vi "Timestamp_Analyzer.vi"() -> ()   [LabVIEW 2020]
uses:
  <vilib>/Analysis/baseanly.llb/Mean (DBL).vi
  <vilib>/Analysis/NI_AALBase.lvlib
panel:
  out "Difference (ns) Standard Deviation":dbl format="%0.2f"
  out "Delta T LLP (ns) Standard Deviation":dbl format="%0.2f"
  out "Delta T LLP (ns) Min":dbl format="%0.2f"
  out "Delta T raw (ns) Standard Deviation":dbl format="%0.2f"
  out "Delta T raw (ns) Min":dbl format="%0.2f"
  out "Difference (ns) Min":dbl format="%0.2f"
  out "Difference (ns) Max":dbl format="%0.2f"
  in  "Timestamp Txt Path":path
  in  "RAW Timestamp from txt File":bool=TRUE
  out "error out":errorcluster
  in  "LLP Timestamp from TDMS File":bool=TRUE
  in  "Timestamp TDMS Path":path
  in  "Skip First N Timestamp":i32=1
  in  "rawdata_Timestamp (ns) type":T1(ring)
  out "Difference (ns) Mean":dbl format="%0.2f"
  out "Delta T LLP (ns) Max":dbl format="%0.2f"
  out "Delta T LLP  (ns) Mean":dbl format="%0.2f"
  out "Delta T raw (ns) Max":dbl format="%0.2f"
  out "Delta T raw (ns) Mean":dbl format="%0.2f"
  out "Difference":dbl[](graph)
  out "Delta T (ns) raw":dbl[](array[numeric])
  out "Delta T (ns) LLP":dbl[](array[numeric])
  out "Size not match":bool
  in  "TDMS LLP Timestamp (s)":dbl[](array[numeric])
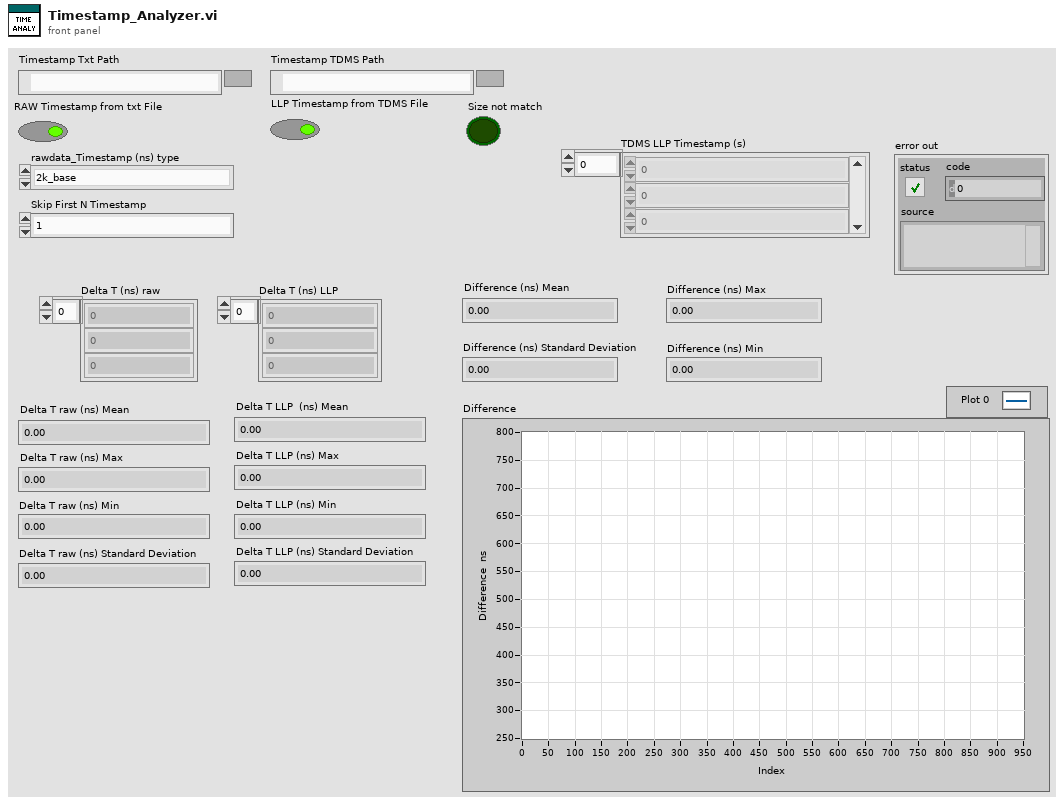
[diagram p1: front panel]
types:
  T1 = enum16{"2k_base", "2k_noise", "4k_base", "4k_noise"}
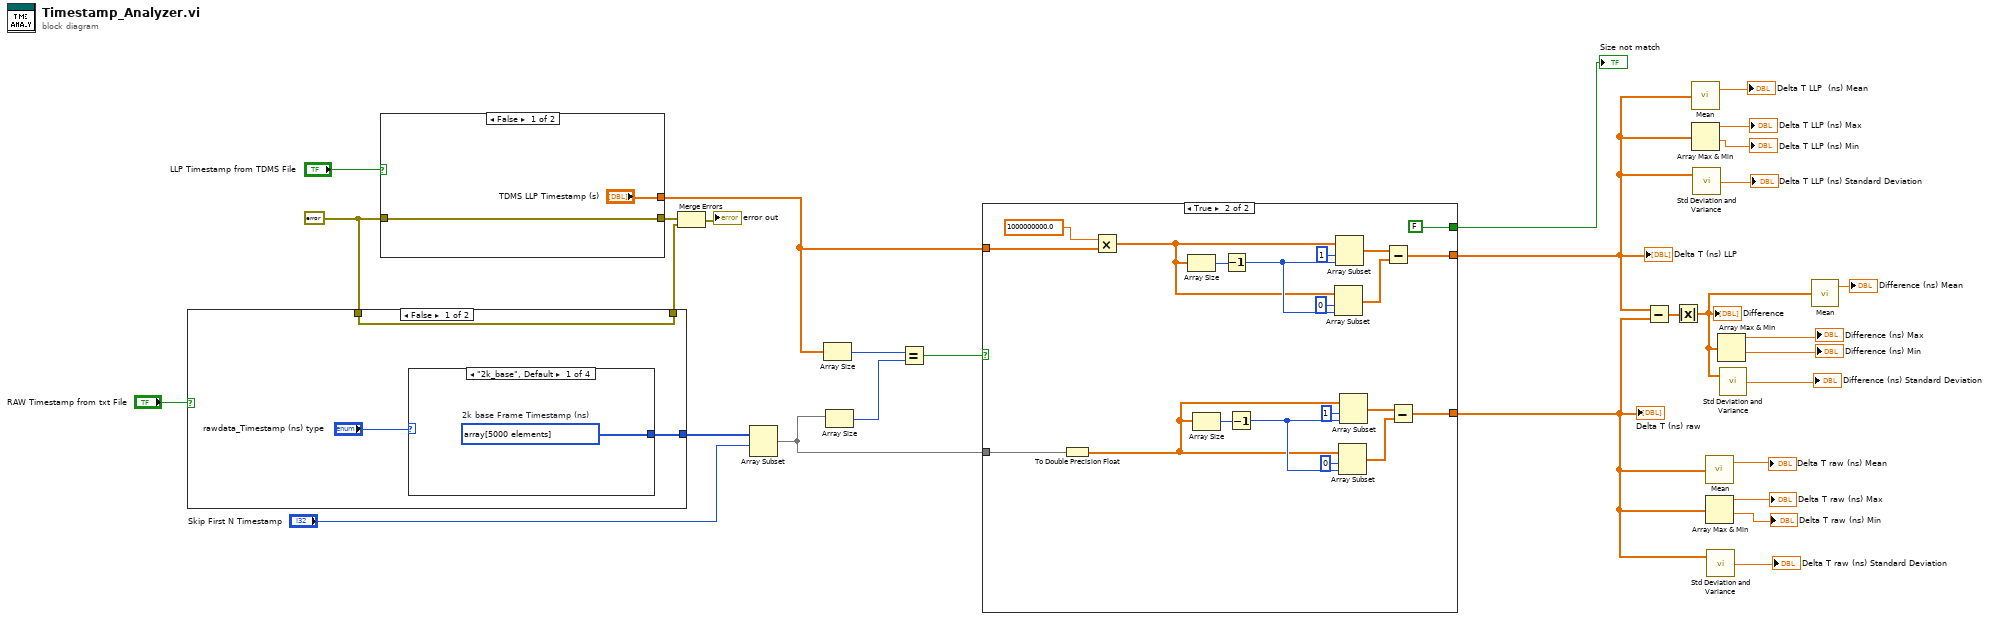
[diagram p0: block diagram]
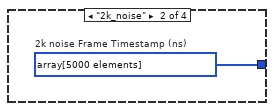
[diagram p2: hidden frame]
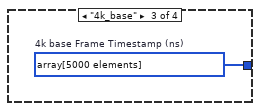
[diagram p3: hidden frame]
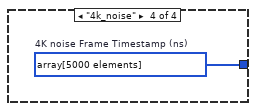
[diagram p4: hidden frame]
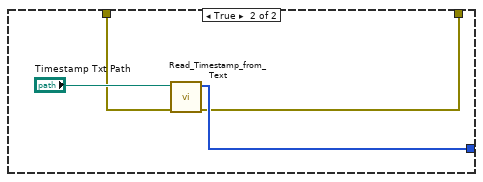
[diagram p5: hidden frame]
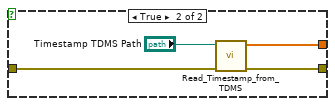
[diagram p6: hidden frame]
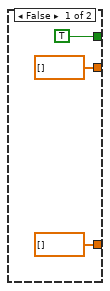
[diagram p7: hidden frame]
diagram:
  w17 = errorcluster {"status"=FALSE, "code"=0, "source"=""} ("error in (no error)")
  n1 = case shown="False" "RAW Timestamp from txt File" {
    tunnel: [w32 w39] -> w21
    tunnel: w17 -> [w31 w40]
    tunnel: [w31 w38] -> w14
    frame False {
      n2 = case shown="\"2k_base\", Default" "rawdata_Timestamp (ns) type" {
        tunnel: [w34 w35 w36 w37] -> w32
        frame "2k_base", Default {
          w34 = u64[] array[5000 elements]  # 2k base Frame Timestamp (ns)
        }
        frame "2k_noise" {
          w35 = u64[] array[5000 elements]  # 2k noise Frame Timestamp (ns)
        }
        frame "4k_base" {
          w36 = u64[] array[5000 elements]  # 4k base Frame Timestamp (ns)
        }
        frame "4k_noise" {
          w37 = u64[] array[5000 elements]  # 4K noise Frame Timestamp (ns)
        }
      }
    }
    frame True {
      n3 = call "Read_Timestamp_from_Text.vi"("error in (no error)"=w40, "Txt File path"="Timestamp Txt Path") -> ("error out"=w38:errorcluster, "relative timestamp (ns)"=w39:u64[])  [unwired: 7 in, 1 out]
    }
  }
  n4 = case shown="False" "LLP Timestamp from TDMS File" {
    tunnel: w17 -> [w43 w46]
    tunnel: ["TDMS LLP Timestamp (s)" w45] -> w19
    tunnel: [w43 w44] -> w16
    frame False {
    }
    frame True {
      n5 = call "Read_Timestamp_from_TDMS.vi"("error in (no error)"=w46, "TDMS File path"="Timestamp TDMS Path") -> ("error out"=w44:errorcluster, "relative timestamp (s)"=w45:dbl[])  [unwired: 7 in, 1 out]
    }
  }
  n6 = Merge Errors(w16, w14) -> (→"error out":errorcluster)
  n7 = Array Subset(array=w21, index="Skip First N Timestamp") -> (w25:u64[])  [unwired: 1 in]
  n8 = Array Size(array=w19) -> (size(s)=w30:i32)
  n9 = Array Size(array=w25) -> (size(s)=w29:i32)
  n10 = Equal?(x=w30, y=w29) -> (x = y?=w28:bool)
  n11 = case shown="True" w28 {
    tunnel: [TRUE ("Size not match") FALSE ("Size not match")] -> w27
    tunnel: w19 -> [_ w69]
    tunnel: [dbl[] [] w61] -> w4
    tunnel: w25 -> [_ w54]
    tunnel: [dbl[] [] w53] -> w8
    frame False {
    }
    frame True {
      n12 = To Double Precision Float(number=w54) -> (double precision float=w51:dbl[])
      n13 = Multiply(x=1000000000.0, y=w69) -> (x*y=w52:dbl[])
      n14 = Array Size(array=w52) -> (size(s)=w67:i32)
      n15 = Array Size(array=w51) -> (size(s)=w60:i32)
      n16 = Decrement(x=w67) -> (x-1=w66:i32)
      n17 = Decrement(x=w60) -> (x-1=w59:i32)
      n18 = Array Subset(array=w52, index=0, length=w66) -> (w62:dbl[])
      n19 = Array Subset(array=w52, index=1, length=w66) -> (w63:dbl[])
      n20 = Array Subset(array=w51, index=0, length=w59) -> (w55:dbl[])
      n21 = Array Subset(array=w51, index=1, length=w59) -> (w56:dbl[])
      n22 = Subtract(x=w63, y=w62) -> (x-y=w61:dbl[])
      n23 = Subtract(x=w56, y=w55) -> (x-y=w53:dbl[])
    }
  }
  "Size not match" <- w27
  "Delta T (ns) LLP" <- w4
  "Delta T (ns) raw" <- w8
  n24 = Subtract(x=w4, y=w8) -> (x-y=w13:dbl[])
  n25 = Absolute Value(x=w13) -> (abs(x)=w2:dbl[])
  "Difference" <- w2
  n26 = call-poly <vilib>:"Mean.vi"("X"=w4) -> ("mean"=→"Delta T LLP  (ns) Mean":dbl)  [unwired: 1 out]
  n27 = Array Max & Min(array=w4) -> (max value=→"Delta T LLP (ns) Max":dbl, min value=→"Delta T LLP (ns) Min":dbl)  [unwired: 2 out]
  n28 = call <vilib>:"Std Deviation and Variance.vi"("X"=w4) -> ("standard deviation"=→"Delta T LLP (ns) Standard Deviation":dbl)  [unwired: 1 in, 2 out]
  n29 = call-poly <vilib>:"Mean.vi"("X"=w8) -> ("mean"=→"Delta T raw (ns) Mean":dbl)  [unwired: 1 out]
  n30 = Array Max & Min(array=w8) -> (max value=→"Delta T raw (ns) Max":dbl, min value=→"Delta T raw (ns) Min":dbl)  [unwired: 2 out]
  n31 = call <vilib>:"Std Deviation and Variance.vi"("X"=w8) -> ("standard deviation"=→"Delta T raw (ns) Standard Deviation":dbl)  [unwired: 1 in, 2 out]
  n32 = Array Max & Min(array=w2) -> (max value=→"Difference (ns) Max":dbl, min value=→"Difference (ns) Min":dbl)  [unwired: 2 out]
  n33 = call <vilib>:"Std Deviation and Variance.vi"("X"=w2) -> ("standard deviation"=→"Difference (ns) Standard Deviation":dbl)  [unwired: 1 in, 2 out]
  n34 = call-poly <vilib>:"Mean.vi"("X"=w2) -> ("mean"=→"Difference (ns) Mean":dbl)  [unwired: 1 out]
